vi "Initialize.vi"(8 "error in (no error)":errorcluster, 10 "Components":refnum<class "1553 Component.lvclass">[](array[class])) -> (0 "error out":errorcluster, 3 "1553 Board out":refnum<class "1553 Session.lvclass">)   [LabVIEW 2020, in "BCI-1553 API.lvlib" / "1553 Session.lvclass"]
doc: "Initializes a 1553 Session with the BCI-1553 hardware. Each Session can have up to 8 components. The total number of available components depends on the number of BCI-1553 modules present."
uses:
  1553 Session.lvclass
  1553 Component/1553 Component.lvclass
  1553 Session.lvclass/1553 Session.ctl
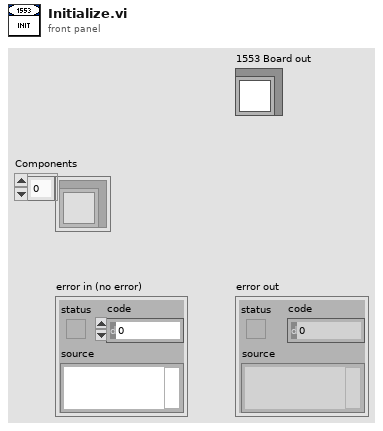
[diagram p1: front panel]
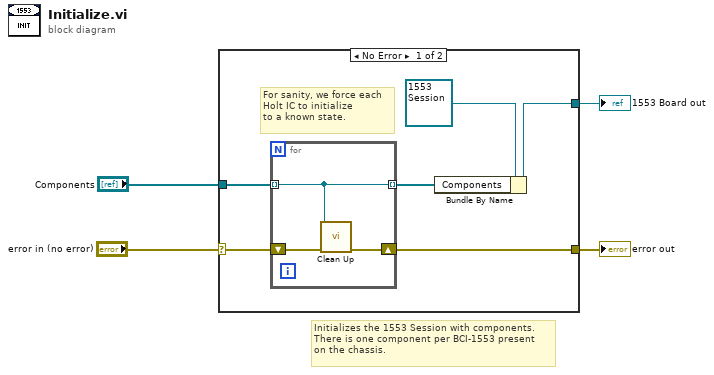
[diagram p0: block diagram]
diagram:
  # "Initializes the 1553 Session with components.\nThere is one component per BCI-1553 present\non the chassis."
  n1 = case shown="No Error" "error in (no error)" {
    selector: "error in (no error)" -> [w8 w14]
    tunnel: [w7 w14] -> w3
    tunnel: [w9 _] -> w2
    tunnel: "Components" -> [w6 _]
    frame No Error {
      # "For sanity, we force each\nHolt IC to initialize\nto a known state."
      n2 = for {
        tunnel: w6 -> [w11] mode=indexing
        tunnel: [w11] -> w5 mode=indexing
        shift-right: [w12] -> w7
        shift-left: w8 -> [w13]
        n3 = call-dynamic "Clean Up.vi"("error in (no error)"=w13, "1553 Component in"=w11) -> ("error out"=w12:errorcluster)  [unwired: 9 in]
      }
      n4 = Bundle By Name(cluster=refnum<class "1553 Session.lvclass"> refnum ("1553 Board out"), "Components"=w5) -> (w9:refnum<class "1553 Session.lvclass">)
    }
    frame Error {
    }
  }
  "error out" <- w3
  "1553 Board out" <- w2
